vi "Filter_Notch50A.vi"(8 "error in (no error)":errorcluster, 9 "Input Data":i32 format="%.0x", 11 "Delay Data":i32[](array[numeric]) format="%.0x") -> (0 "error out":errorcluster, 1 "Filtered Data":i32 format="%.0x", 2 "Node Data out":i32[](array[numeric]) format="%.0x", 3 "Delay Data out":i32[](array[numeric]) format="%.0x")   [LabVIEW 2010]
doc: "This VI implements the first of two cascaded, 2nd order, IIR, digital 50Hz notch filter on the input data.\nThe input data should be at a data rate = 500SPS. The data is filtered point-by-point.\n\nInputs:\nInput Data - (I32[]) data @ 500SPS to be filtered\nDelay Data - (I32[]) previous array values used in digital filtering\nerror in - error input cluster\n\nOutputs:\nFilter Data - (I32[]) data @ 500SPS filtered\nDelay Data out - (I32[]) previous array values used in digital filtering to pass to next filter stage\nNode Data out - (I32[]) node data to pass to next filter stage\nerror out - error output cluster"
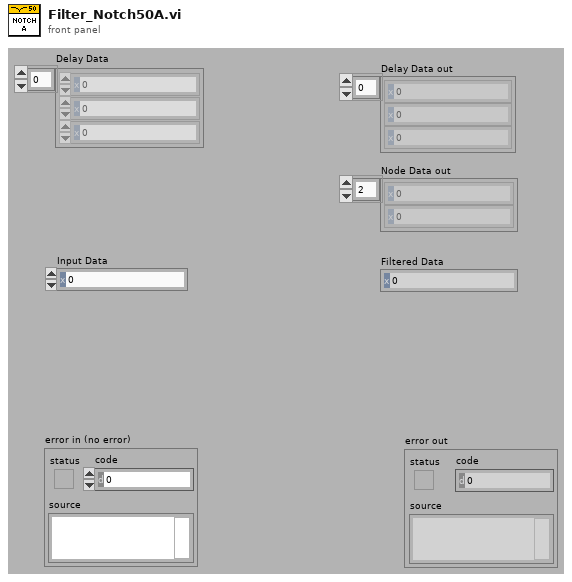
[diagram p1: front panel]
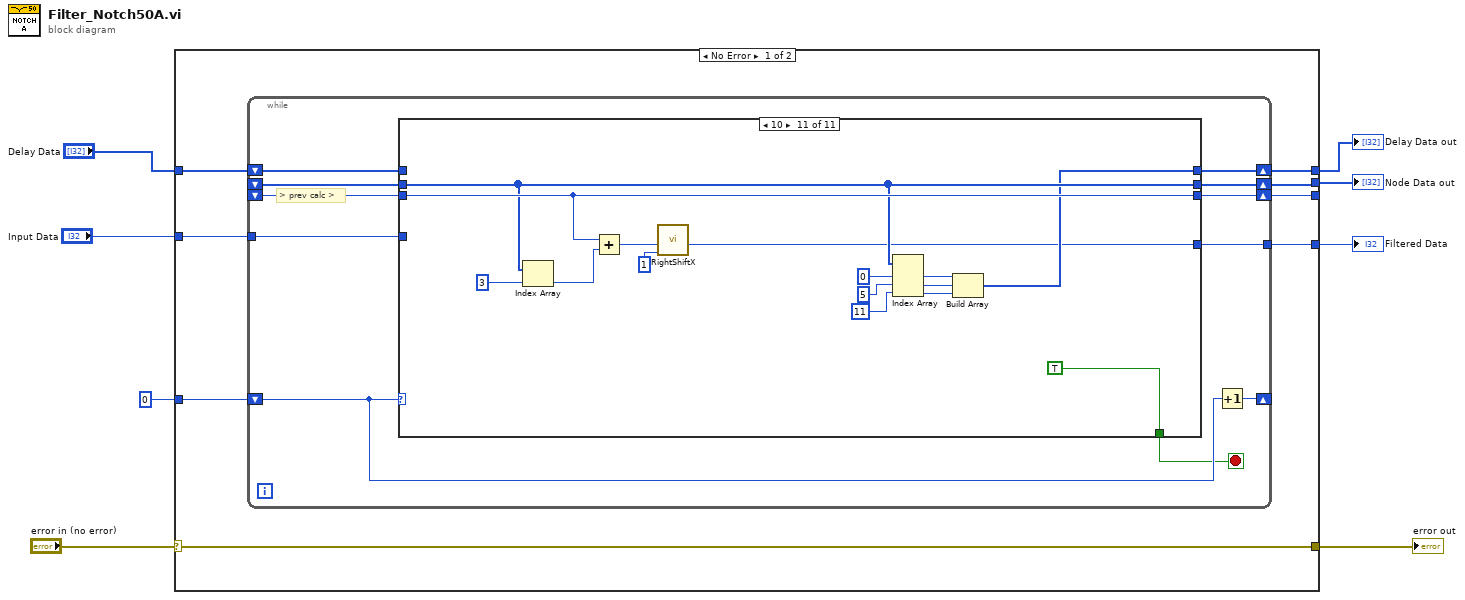
[diagram p0: block diagram]
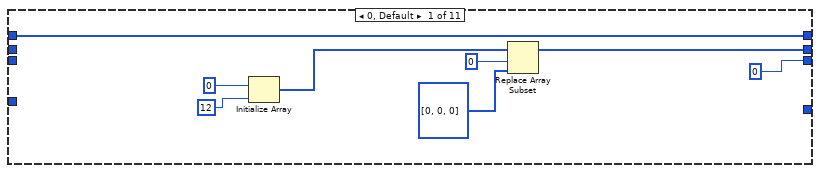
[diagram p2: hidden frame]
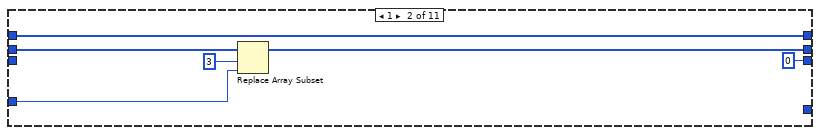
[diagram p3: hidden frame]
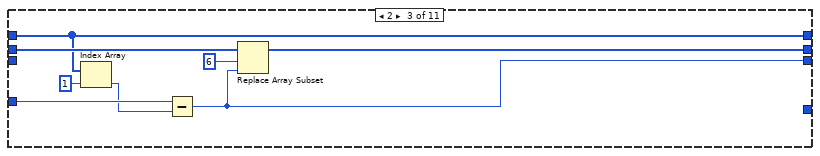
[diagram p4: hidden frame]
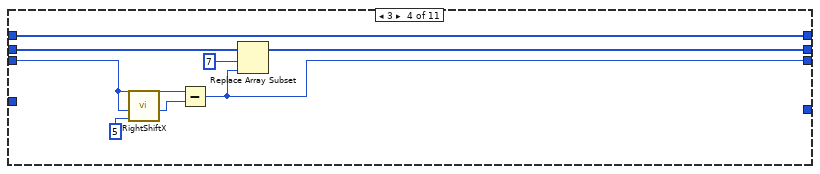
[diagram p5: hidden frame]
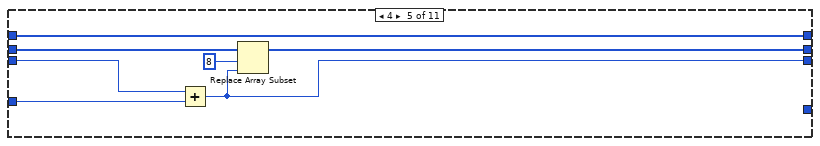
[diagram p6: hidden frame]
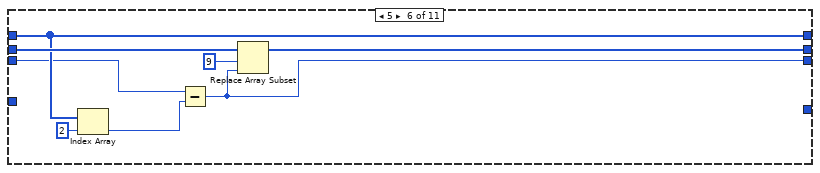
[diagram p7: hidden frame]
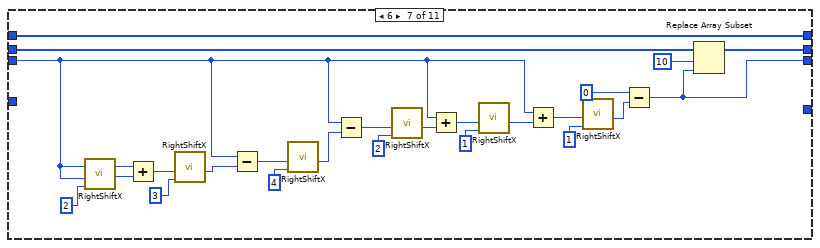
[diagram p8: hidden frame]
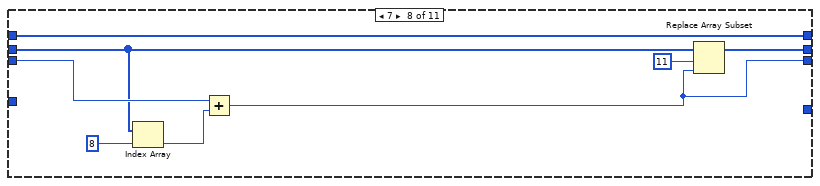
[diagram p9: hidden frame]
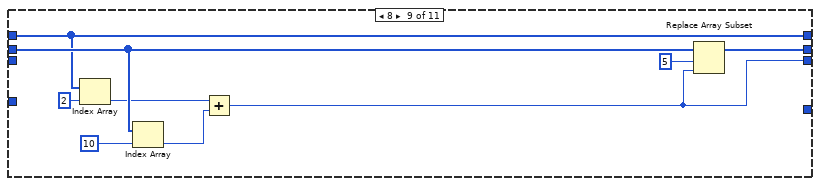
[diagram p10: hidden frame]
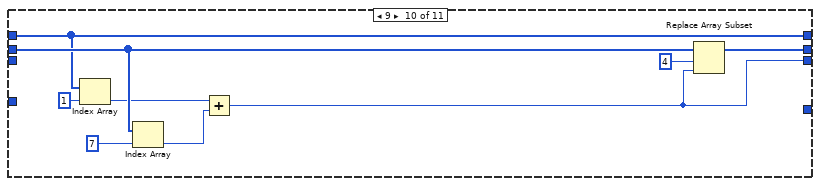
[diagram p11: hidden frame]
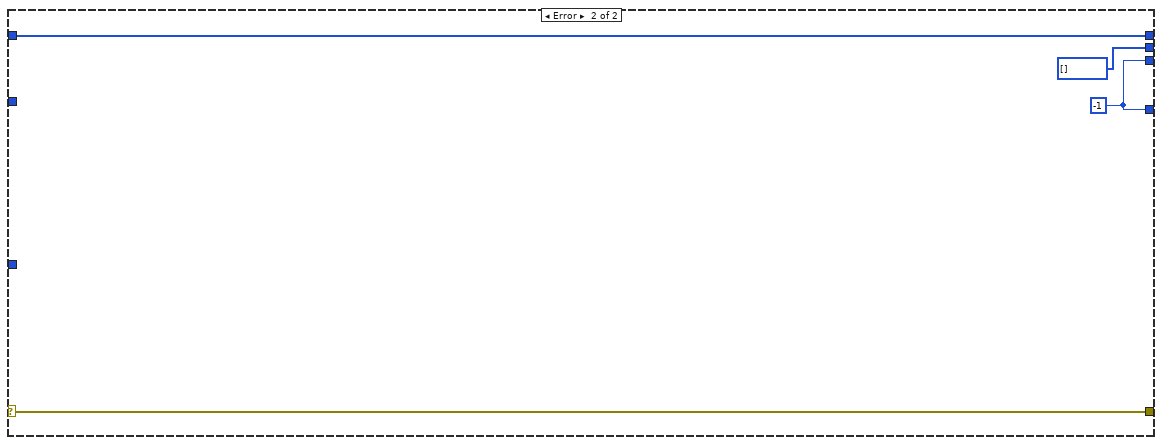
[diagram p12: hidden frame]
diagram:
  n1 = case shown="No Error" "error in (no error)" {
    selector: "error in (no error)" -> [w9 w141]
    tunnel: [w9 w141] -> w7
    tunnel: [w16 w140] -> w1
    tunnel: [w15 i32[] []] -> w2
    tunnel: 0 -> [w14 _]
    tunnel: "Input Data" -> [w13 _]
    tunnel: "Delay Data" -> [w12 w140]
    tunnel: [w11 w139] -> _
    tunnel: [w10 w139] -> w3
    frame No Error {
      n2 = while {
        shift-right: [w26] -> w15
        shift-left: _ -> [w25]
        shift-right: [w24] -> _
        shift-left: w14 -> [w23]
        tunnel: w13 -> [w22]
        shift-right: [w27] -> w16
        shift-left: w12 -> [w21]
        shift-right: [w19] -> w11
        shift-left: _ -> [w18]
        tunnel: [w17] -> w10
        stop <- w20 stop-if-true
        # "> prev calc >"
        n3 = case shown="10" w23 {
          tunnel: [w32 w38 w45 w55 w62 w68 w94 w102 w107 w116 w126] -> w27
          tunnel: [w35 w39 w47 w57 w64 w72 w96 w104 w113 w122 w133] -> w26
          tunnel: w25 -> [_ w41 w49 w54 w60 w70 w92 w100 w111 w120 w133]
          tunnel: w22 -> [_ w40 w48 _ w61 _ _ _ _ _ _]
          tunnel: w21 -> [w32 w38 w45 w55 w62 w68 w94 w102 w107 w116 _]
          tunnel: [_ _ _ _ _ _ _ _ _ _ TRUE] -> w20
          tunnel: [0 0 w42 w53 w59 w65 w91 w97 w109 w118 w134] -> w19
          tunnel: w18 -> [_ _ _ w51 w58 w66 w73 w101 _ _ w134]
          tunnel: [_ _ _ _ _ _ _ _ _ _ w123] -> w17
          frame 0, Default {
            n4 = Initialize Array(0 ("index"), 12 ("index")) -> (w28:i32[])
            n5 = Replace Array Subset(array=w28, new element=i32[] [0, 0, 0] ("Node Data"), index=0) -> (w35:i32[])
          }
          frame 1 {
            n6 = Replace Array Subset(array=w41, new element=w40, index=3) -> (w39:i32[])
          }
          frame 2 {
            n7 = Index Array(array=w45, index=1) -> (element=w43:i32)
            n8 = Subtract(x=w48, y=w43) -> (x-y=w42:i32)
            n9 = Replace Array Subset(array=w49, new element=w42, index=6) -> (w47:i32[])
          }
          frame 3 {
            n10 = call "RightShiftX.vi"("Shift"=i8 5 ("y"), "Data"=w51) -> ("Shifted Data"=w50:i32)  [unwired: 9 out]
            n11 = Subtract(x=w51, y=w50) -> (x-y=w53:i32)
            n12 = Replace Array Subset(array=w54, new element=w53, index=7) -> (w57:i32[])
          }
          frame 4 {
            n13 = Add(x=w58, y=w61) -> (x+y=w59:i32)
            n14 = Replace Array Subset(array=w60, new element=w59, index=8) -> (w64:i32[])
          }
          frame 5 {
            n15 = Index Array(array=w68, index=2) -> (element=w67:i32)
            n16 = Subtract(x=w66, y=w67) -> (x-y=w65:i32)
            n17 = Replace Array Subset(array=w70, new element=w65, index=9) -> (w72:i32[])
          }
          frame 6 {
            n18 = call "RightShiftX.vi"("Shift"=i8 2 ("y"), "Data"=w73) -> ("Shifted Data"=w88:i32)  [unwired: 9 out]
            n19 = Add(x=w73, y=w88) -> (x+y=w89:i32)
            n20 = call "RightShiftX.vi"("Shift"=i8 3 ("y"), "Data"=w89) -> ("Shifted Data"=w86:i32)  [unwired: 9 out]
            n21 = Subtract(x=w73, y=w86) -> (x-y=w85:i32)
            n22 = call "RightShiftX.vi"("Shift"=i8 4 ("y"), "Data"=w85) -> ("Shifted Data"=w77:i32)  [unwired: 9 out]
            n23 = Subtract(x=w73, y=w77) -> (x-y=w78:i32)
            n24 = call "RightShiftX.vi"("Shift"=i8 2 ("y"), "Data"=w78) -> ("Shifted Data"=w76:i32)  [unwired: 9 out]
            n25 = Add(x=w73, y=w76) -> (x+y=w75:i32)
            n26 = call "RightShiftX.vi"("Shift"=i8 1 ("y"), "Data"=w75) -> ("Shifted Data"=w80:i32)  [unwired: 9 out]
            n27 = Add(x=w73, y=w80) -> (x+y=w74:i32)
            n28 = call "RightShiftX.vi"("Shift"=i8 1 ("y"), "Data"=w74) -> ("Shifted Data"=w82:i32)  [unwired: 9 out]
            n29 = Subtract(x=0 ("index"), y=w82) -> (x-y=w91:i32)
            n30 = Replace Array Subset(array=w92, new element=w91, index=10) -> (w96:i32[])
          }
          frame 7 {
            n31 = Index Array(array=w100, index=8) -> (element=w98:i32)
            n32 = Add(x=w101, y=w98) -> (x+y=w97:i32)
            n33 = Replace Array Subset(array=w100, new element=w97, index=11) -> (w104:i32[])
          }
          frame 8 {
            n34 = Index Array(array=w107, index=2) -> (element=w105:i32)
            n35 = Index Array(array=w111, index=10) -> (element=w110:i32)
            n36 = Add(x=w105, y=w110) -> (x+y=w109:i32)
            n37 = Replace Array Subset(array=w111, new element=w109, index=5) -> (w113:i32[])
          }
          frame 9 {
            n38 = Index Array(array=w116, index=1) -> (element=w114:i32)
            n39 = Index Array(array=w120, index=7) -> (element=w119:i32)
            n40 = Add(x=w114, y=w119) -> (x+y=w118:i32)
            n41 = Replace Array Subset(array=w120, new element=w118, index=4) -> (w122:i32[])
          }
          frame 10 {
            n42 = Index Array(array=w133, index=3) -> (element=w136:i32)
            n43 = Add(x=w134, y=w136) -> (x+y=w124:i32)
            n44 = call "RightShiftX.vi"("Shift"=i8 1 ("y"), "Data"=w124) -> ("Shifted Data"=w123:i32)  [unwired: 9 out]
            n45 = Index Array(array=w133, index #1=0 ("index"), index #2=5 ("index"), index #3=11 ("index")) -> (element #1=w129:i32, element #2=w128:i32, element #3=w127:i32)
            n46 = Build Array(w129, w128, w127) -> (w126:i32[])
          }
        }
        n47 = Increment(x=w23) -> (x+1=w24:i32)
      }
    }
    frame Error {
      w139 = -1
    }
  }
  "error out" <- w7
  "Filtered Data" <- w3
  "Node Data out" <- w2
  "Delay Data out" <- w1
